vi "Standard Engine.vi"(8 "error in":errorcluster, 11 "Engine Process Init Data":T1) -> (0 "error out":errorcluster)   [LabVIEW 2013, in "Standard Engine Runtime.lvclass"]
doc: "This VI is a process that executes modules and has an API for transitioning through its state machine. Once it is initialized and running, it calls an array of module input methods, followed by an array of module process methods, followed by an array of module output methods, and then does any necessary error handling and bookkeeping."
uses:
  Standard Engine Runtime.lvclass
  Engine Process Init Data.ctl
  Commands.ctl
  Engine Config Data.ctl
  Configuration/Standard Engine Configuration.lvclass
  <vilib>/NI/Tag Bus Module Framework/runtime/TBM module execution interface.lvclass
  <vilib>/NI/Tag Bus Module Framework/module configuration/TBM module configuration.lvclass
  <vilib>/NI/Module Execution Interface/Engine Runtime/Execution States.ctl
  Engine Data.ctl
  Configuration/Loop Info.ctl
  <vilib>/NI/Tag Bus/table/data table.ctl
  Module Execution Info.ctl
  Data Table with Transfer Spec.ctl
  <vilib>/NI/Tag Bus/table/transfer specification.ctl
  <vilib>/NI/Tag Bus/tag/Data Type.ctl
  Configuration/Module Decimation.ctl
  Configuration/Module Error Configuration.ctl
  Configuration/Error Actions By Category.ctl
  <vilib>/NI/Tag Bus Module Framework/runtime/error classification.ctl
  Configuration/Error Actions.ctl
  <vilib>/NI/Module Timing Source/timing source/TBM timing source.lvclass
  Configuration/timing policy.ctl
  async execution info.ctl
  asynchronous process data.ctl
  async command notification.ctl
  <vilib>/NI/Tag Bus Module Framework/runtime/execution settings.ctl
  async error info.ctl
  status reporting data.ctl
  module status reporting.ctl
  <vilib>/Platform/TimedLoop/XDataNode/timing_clust.ctl
  <vilib>/Platform/TimedLoop/XDataNode/nitl_modes.ctl
  <vilib>/Platform/TimedLoop/XDataNode/wakeup.ctl
  <vilib>/NI/Tag Bus/table/transfer table data.vi
  Module Execution Decimation.vi
  Error Handler.vi
  <vilib>/NI/Tag Bus/table/write data element.vi
  <vilib>/NI/Tag Bus/table/data polymorphs/write one/write Boolean.vi
  <vilib>/NI/Tag Bus/table/data polymorphs/write one/write U32.vi
  <vilib>/NI/Tag Bus/table/data polymorphs/write one/write U64.vi
  <vilib>/NI/Tag Bus/table/data polymorphs/write one/write I32.vi
  Delete Module Index.vi
  <vilib>/platform/TimedLoop/XDataNode/XDataNode.xnode
  <vilib>/NI/Module Execution Interface/Engine Runtime/Engine Runtime Interface.lvclass
  <vilib>/NI/Tag Bus/table/data table.lvlib
  <vilib>/NI/Tag Bus/tag/tag descriptor.lvclass
  <vilib>/Platform/TimedLoop/XDataNode/XDNodeRunTimeDep.lvlib
panel:
  out "iterations":i32
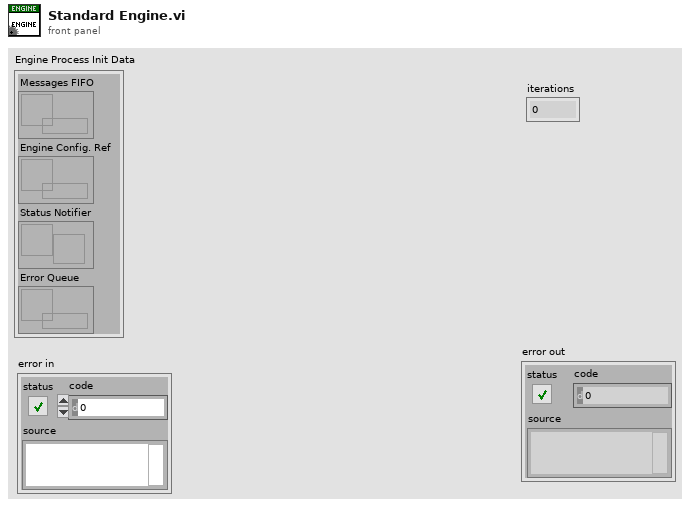
[diagram p1: front panel]
types:
  T1 = typedef "Standard Engine Runtime.lvclass/Engine Process Init Data.ctl" = cluster{"Messages FIFO":refnum<k33>, "Engine Config. Ref":refnum<data-value>, "Status Notifier":refnum<notifier>, "Error Queue":refnum<queue>}
  T2 = typedef "Standard Engine Runtime.lvclass/Engine Data.ctl" = cluster{"Loop Info":T3, "Main Tag Data":T4, "Module Info":T5, "engine timing source":refnum<class "TBM timing source.lvclass">, "timing policy":T14, "async execution info":T15, "status reporting":T18, "Timing Source dt":u32}
  T3 = typedef "Standard Engine Configuration.lvclass/Loop Info.ctl" = cluster{"Processor":i32, "Priority":i32}
  T4 = typedef "tag bus.lvlib/data table.lvlib/data table.ctl" = cluster{"Double":dbl[], "Single":sgl[], "I64":i64[], "I32":i32[], "I16":i16[], "I8":i8[], "U64":u64[], "U32":u32[], "U16":u16[], "U8":u8[], "Boolean":bool[], "String":string[], "Array of Double":cluster{"DBL Array":dbl[]}[], "Array of Single":cluster{"SGL Array":sgl[]}[], "Array of I64":cluster{"I64 Array":i64[]}[], "Array of I32":cluster{"I32 Array":i32[]}[], "Array of I16":cluster{"I16 Array":i16[]}[], "Array of I8":cluster{"I8 Array":i8[]}[], "Array of U64":cluster{"U64 Array":u64[]}[], "Array of U32":cluster{"U32 Array":u32[]}[], "Array of U16":cluster{"U16 Array":u16[]}[], "Array of U8":cluster{"U8 Array":u8[]}[], "Array of Boolean":cluster{"Boolean Array":bool[]}[], "Array of String":cluster{"String Array":string[]}[]}
  T5 = typedef "Standard Engine Runtime.lvclass/Module Execution Info.ctl" = cluster{"Tag Bus Modules":refnum<class "TBM module execution interface.lvclass">[], "Execute?":bool[], "Input Method Indices":i32[], "Process Method Indices":i32[], "Output Method Indices":i32[], "Input Transfer Specifications":T6[], "Parameter Transfer Specifications":T6[], "Result Transfer Specifications":T6[], "Output Transfer Specifications":T6[], "Module Errors":errorcluster[], "Module Decimation":T9[], "Module Decimation Indices":i32[], "Error Queue":refnum<queue>, "Module Error Configuration":T10[], "Module Errors (n-1)":errorcluster[]}
  T6 = typedef "Standard Engine Runtime.lvclass/Data Table with Transfer Spec.ctl" = cluster{"Data Table":T4, "Transfer Specification":T7[]}
  T7 = typedef "tag bus.lvlib/data table.lvlib/transfer specification.ctl" = cluster{"data type":T8, "sink indices":i32[], "source indices":i32[]}
  T8 = typedef "tag bus.lvlib/tag descriptor.lvclass/Data Type.ctl" = enum16{"Double", "Single", "I64", "I32", "I16", "I8", "U64", "U32", "U16", "U8", "Boolean", "String", "Array of Double", "Array of Single", "Array of I64", "Array of I32", "Array of I16", "Array of I8", "Array of U64", "Array of U32", "Array of U16", "Array of U8", "Array of Boolean", "Array of String"}
  T9 = typedef "Standard Engine Configuration.lvclass/Module Decimation.ctl" = cluster{"Decimation":u16, "Offset":u16}
  T10 = typedef "Standard Engine Configuration.lvclass/Module Error Configuration.ctl" = cluster{"Module Error Configuration":T11[]}
  T11 = typedef "Standard Engine Configuration.lvclass/Error Actions By Category.ctl" = cluster{"error classification":T12, "Error Actions":T13[]}
  T12 = typedef "TBM module execution interface.lvclass/error classification.ctl" = enum16{"unknown", "none", "trivial", "recoverable", "critical"}
  T13 = typedef "Standard Engine Configuration.lvclass/Error Actions.ctl" = enum16{"Clear", "Notify", "Stop Component", "Stop Engine", "Safe State", "Attempt Recovery"}
  T14 = typedef "Standard Engine Configuration.lvclass/timing policy.ctl" = enum16{"strict determinism", "nonblocking", "nondeterministic inline"}
  T15 = typedef "Standard Engine Runtime.lvclass/async execution info.ctl" = cluster{"Tag Bus Modules":T16[], "Execute?":bool[], "Input Method Indices":i32[], "Process Method Indices":i32[], "Output Method Indices":i32[], "Input Transfer Specifications":T6[], "Parameter Transfer Specifications":T6[], "Result Transfer Specifications":T6[], "Output Transfer Specifications":T6[], "Module Errors":errorcluster[], "Module Decimation":T9[], "Module Decimation Indices":i32[], "Error Queue":refnum<queue>, "Module Error Configuration":T10[], "comm errors":errorcluster[]}
  T16 = typedef "Standard Engine Runtime.lvclass/asynchronous process data.ctl" = cluster{"thread reference":refnum<vi>, "cmd notification":refnum<k33>, "execution period (ms)":i32, "input from component":refnum<queue>, "input to component":refnum<queue>, "output from component":refnum<queue>, "output to component":refnum<queue>, "process input from component":refnum<queue>, "process input to component":refnum<queue>, "process result from component":refnum<queue>, "process result to component":refnum<queue>, "execution settings":T17, "error fifo":refnum<k33>}
  T17 = typedef "TBM module execution interface.lvclass/execution settings.ctl" = cluster{"reads inputs":bool, "processes data":bool, "writes outputs":bool}
  T18 = typedef "Standard Engine Runtime.lvclass/status reporting data.ctl" = cluster{"late index (bool)":i32, "late count (U32)":i32, "current dt ns(U64)":i32, "synchronous modules":T19[], "asynchronous modules":T19[]}
  T19 = typedef "Standard Engine Runtime.lvclass/module status reporting.ctl" = cluster{"module index":i32, "error tag (I32)":i32}
  T20 = typedef "Engine Runtime Interface.lvclass/Execution States.ctl" = enum16{"Initializing", "Paused (Initialized)", "Running", "Set Safe Outputs", "Uninitializing", "Stopped (Uninitialized)", "Error (Uninitialized)", "Safe State (Uninitialized)", "Closed"}
  T21 = typedef "Standard Engine Runtime.lvclass/Commands.ctl" = enum16{"Initialize", "Start", "Pause", "Safe State", "Normal", "Stop", "Shutdown"}
  T22 = typedef "XDNodeRunTimeDep.lvlib/timing_clust.ctl" = cluster{"Expected End [f-1]":u64, "Actual End [f-1]":u64, "Finished Late? [f-1]":bool, "Expected End [i-1]":u64, "Actual End [i-1]":u64, "Finished Late? [i-1]":bool, "Expected Start [i]":u64, "Actual Start [i]":u64, "Expected Start [f]":u64, "Actual Start [f]":u64, "Source Name":string, "Structure Name":string, "Period":i64, "Deadline":i64, "Offset":i64, "Start":i64, "Priority":i32, "Timeout":i32, "Mode":T23, "Wakeup Reason":T24, "Error":errorcluster, "Source Type":string, "Secondary Source Type":string, "Global End Time":u64, "Global Start Time":u64, "Frame Duration":u64, "Iteration Duration":u64, "Assigned CPU":i32, "I/O Scan Engine Mode":u32}
  T23 = typedef "XDNodeRunTimeDep.lvlib/nitl_modes.ctl" = enum32{"No Change", "Process missed periods, maintain original phase", "Discard missed periods, maintain original phase", "Process missed periods, ignore original phase", "Discard missed periods, ignore original phase"}
  T24 = typedef "XDNodeRunTimeDep.lvlib/wakeup.ctl" = enum32{"Normal", "Aborted", "Asynchronous wakeup", "Timing source error", "Timed loop error", "Timeout"}
  T25 = typedef "Standard Engine Runtime.lvclass/Engine Config Data.ctl" = cluster{"Engine Configuration":refnum<class "Standard Engine Configuration.lvclass">, "Modules":refnum<class "TBM module execution interface.lvclass">[], "Module Configurations":refnum<class "TBM module configuration.lvclass">[]}
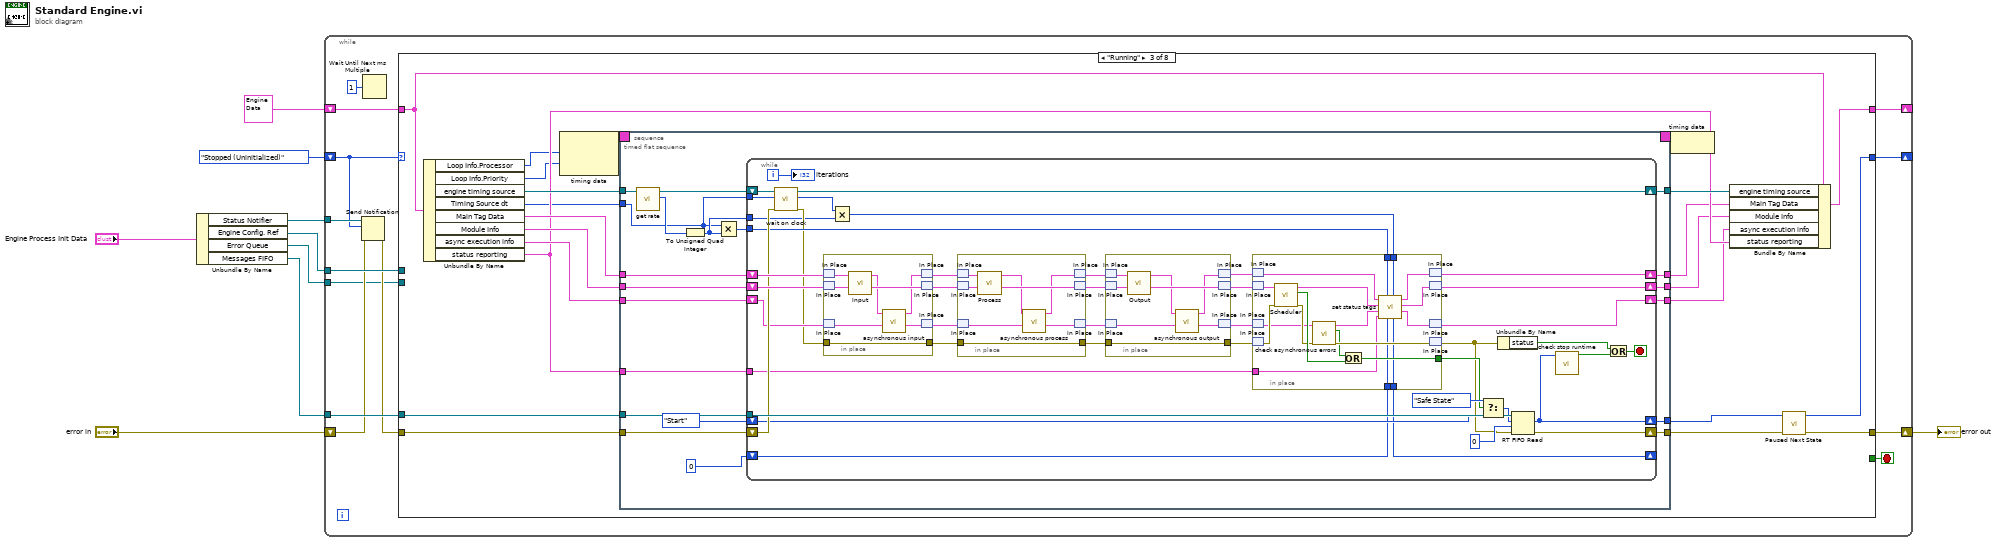
[diagram p0: block diagram]
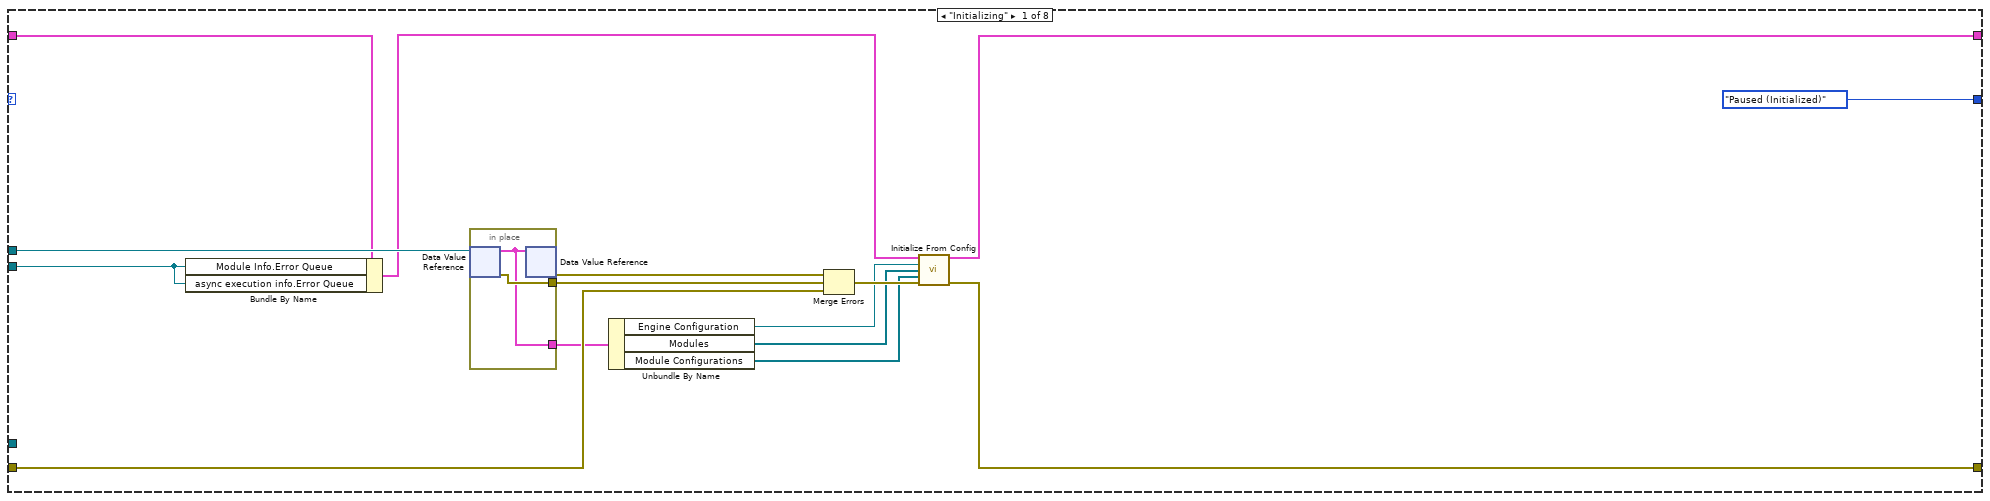
[diagram p2: hidden frame]
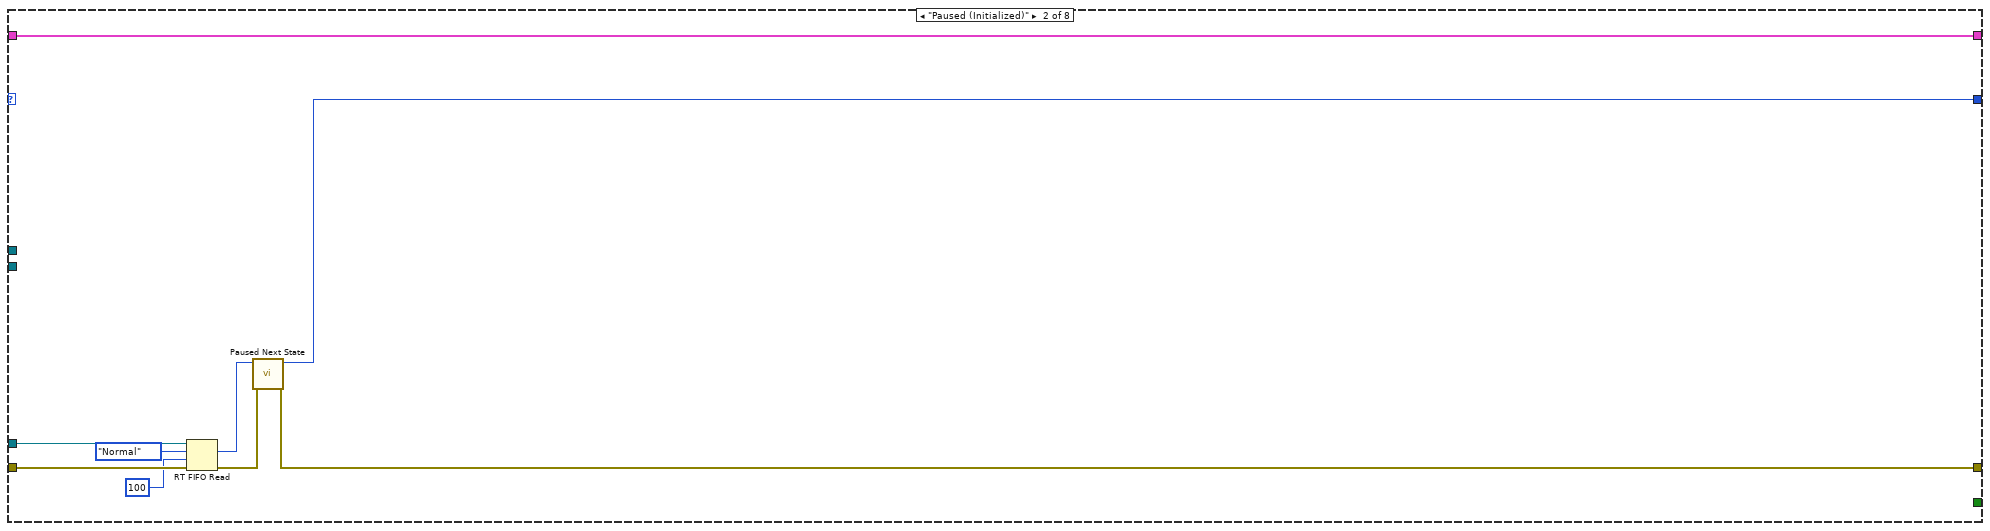
[diagram p3: hidden frame]
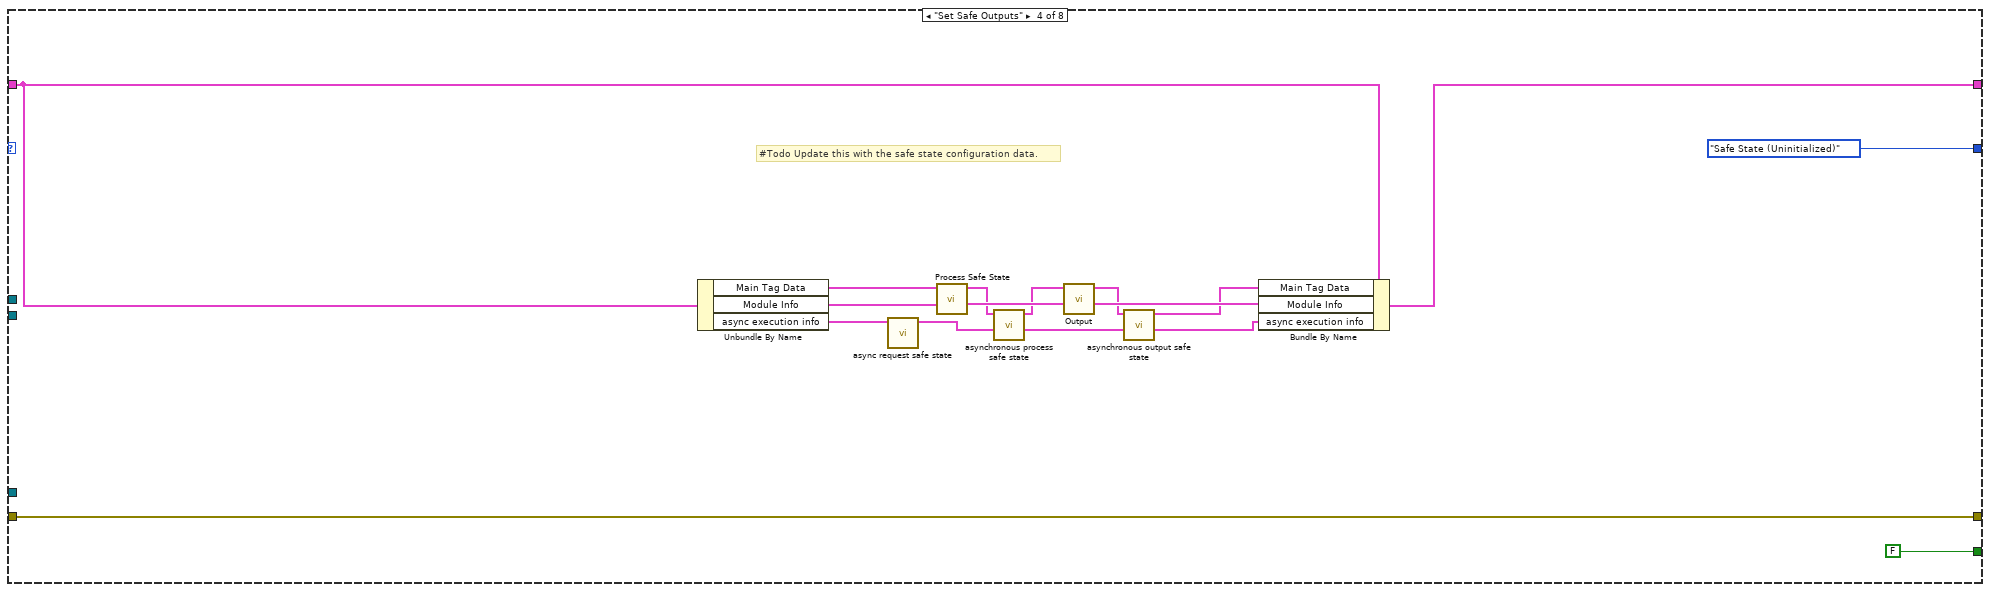
[diagram p4: hidden frame]
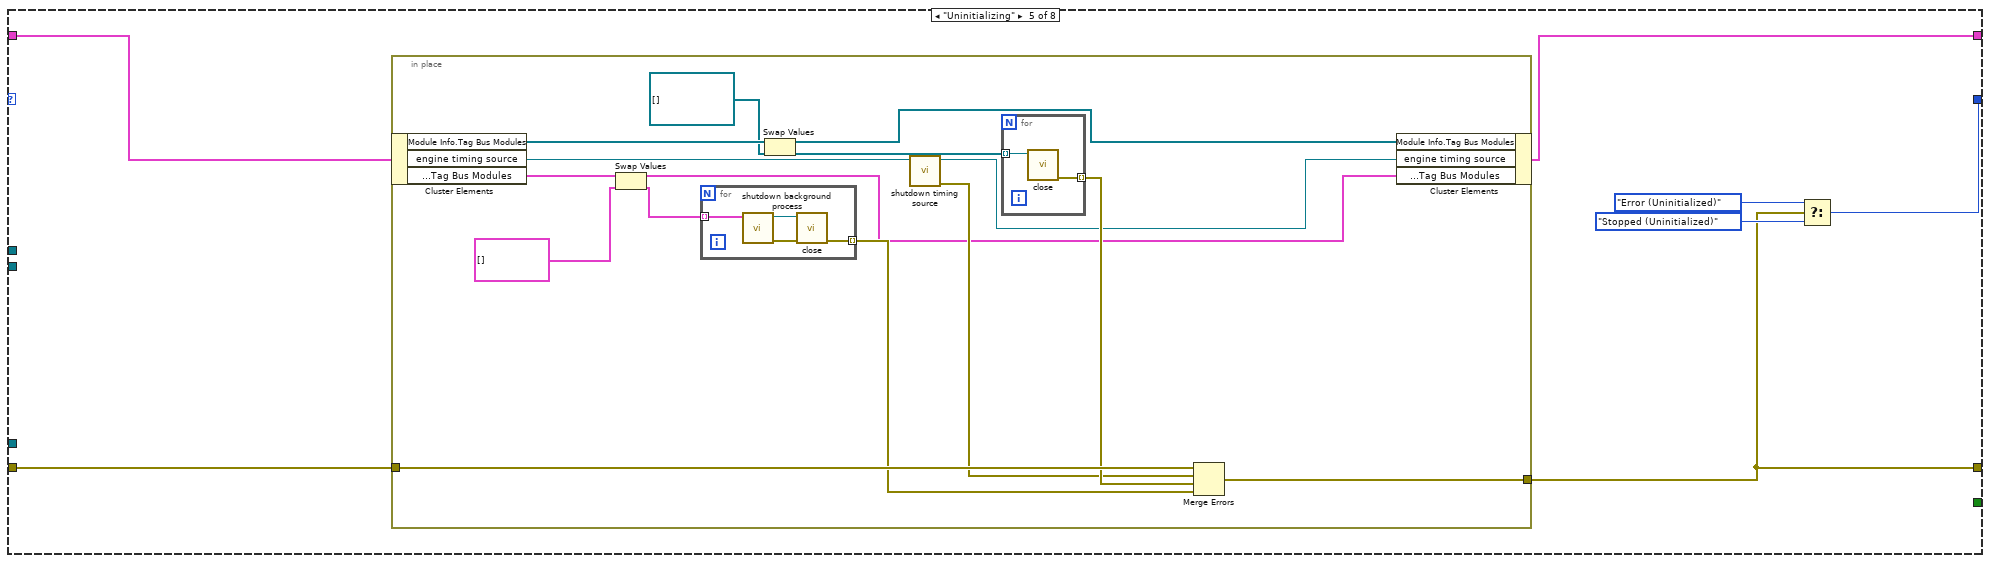
[diagram p5: hidden frame]
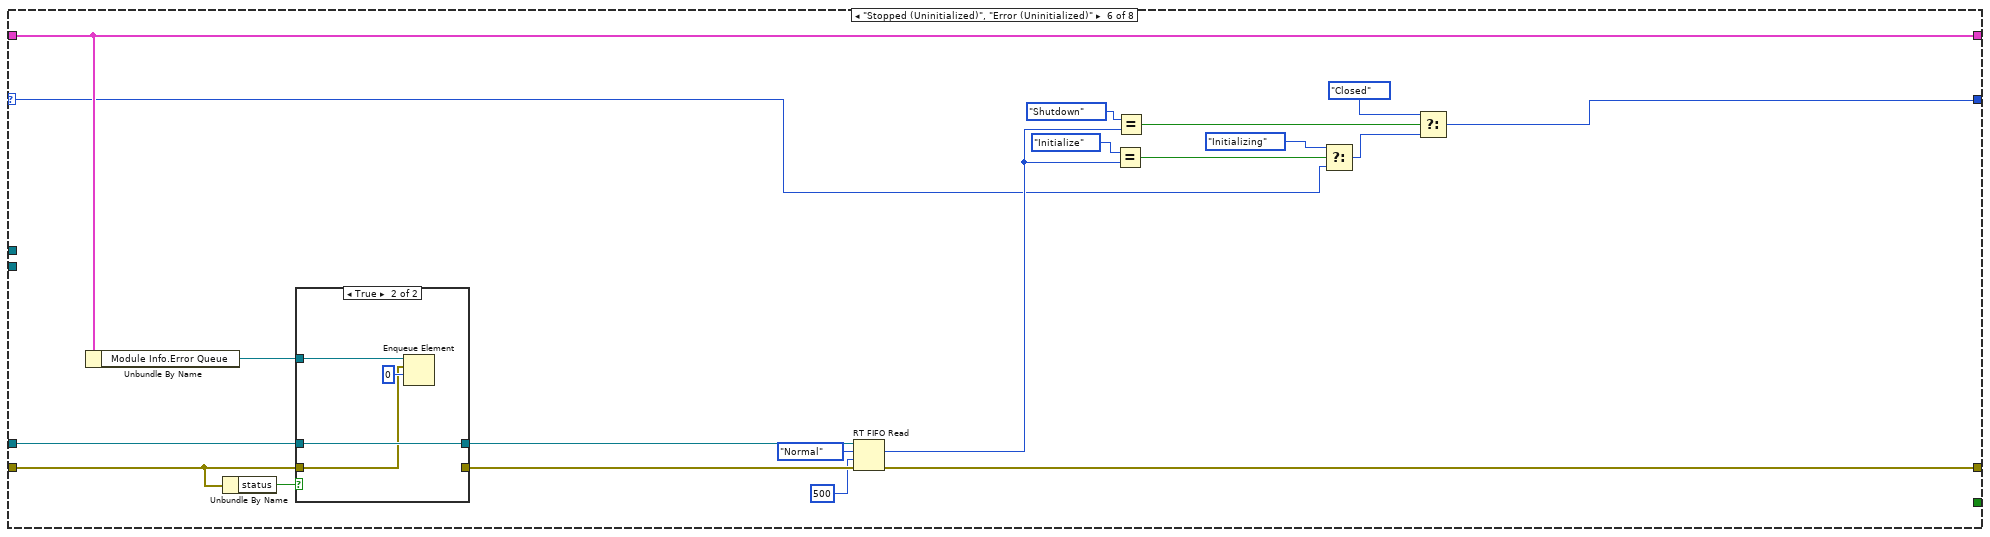
[diagram p6: hidden frame]
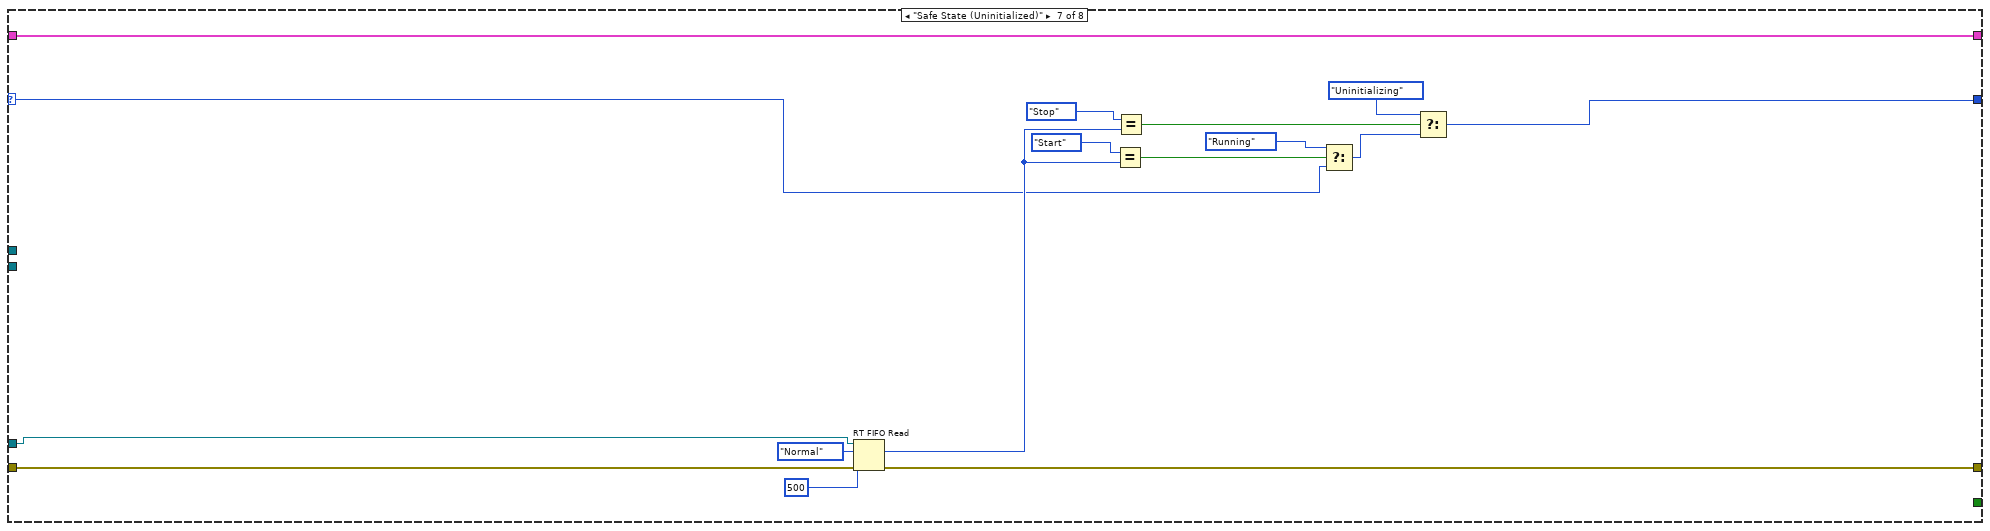
[diagram p8: hidden frame]
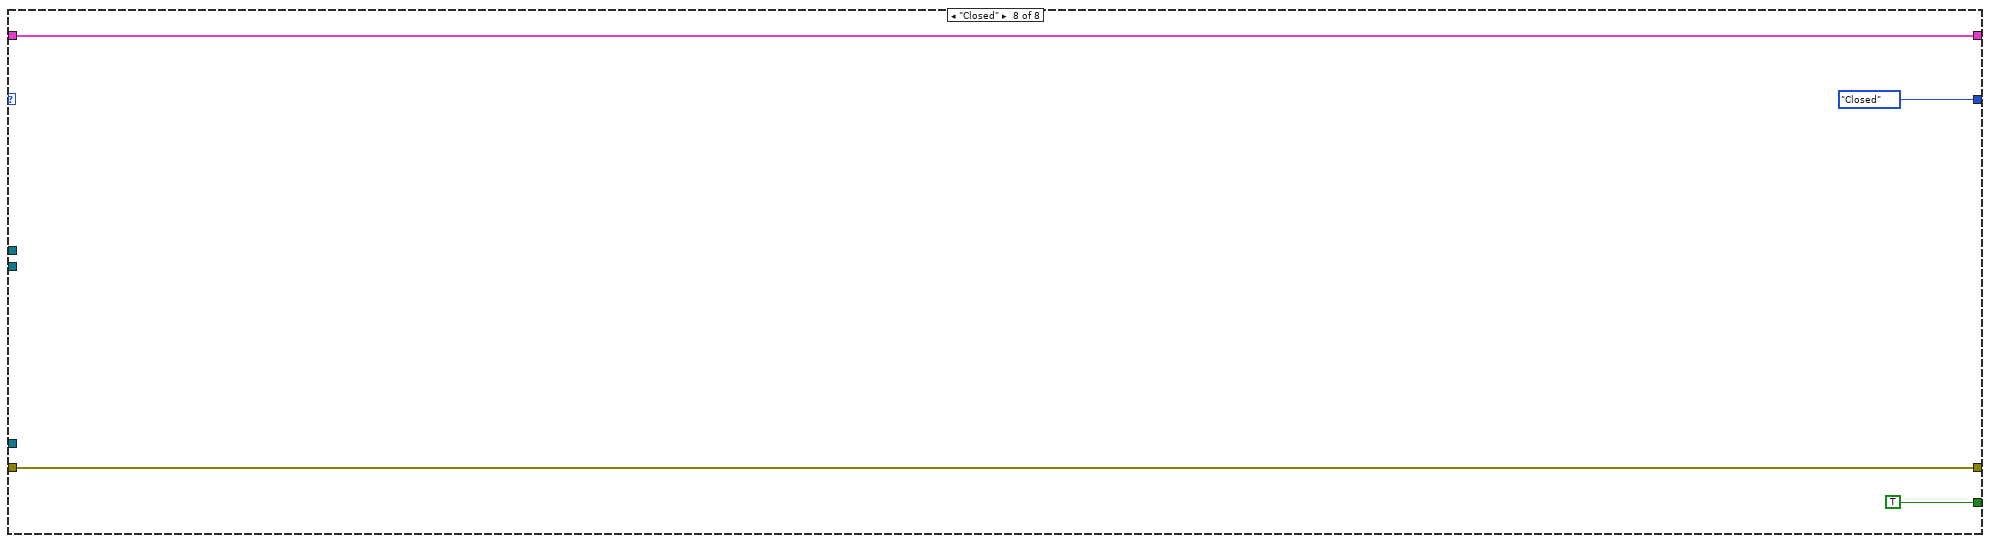
[diagram p9: hidden frame]
diagram:
  n1 = Unbundle By Name("Engine Process Init Data") -> ("Status Notifier"=w7:refnum<notifier>, "Engine Config. Ref"=w6:refnum<data-value>, "Error Queue"=w3:refnum<queue>, "Messages FIFO"=w5:refnum<k33>)
  n2 = while {
    shift-right: [w19] -> _
    shift-left: Execution_States."Stopped (Uninitialized)" ("States") -> [w14]
    shift-right: [w20] -> _
    shift-left: T2 {"Loop Info"={"Processor"=-2, "Priority"=0}, "Main Tag Data"={"Double"=[], "Single"=[], "I64"=[], "I32"=[], "I16"=[], "I8"=[], "U64"=[], "U32"=[], "U16"=[], "U8"=[], "Boolean"=[], "String"=[], "Array of Double"=[], "Array of Single"=[], "Array of I64"=[], "Array of I32"=[], "Array of I16"=[], "Array of I8"=[], "Array of U64"=[], "Array of U32"=[], "Array of U16"=[], "Array of U8"=[], "Array of Boolean"=[], "Array of String"=[]}, "Module Info"={"Tag Bus Modules"=[], "Execute?"=[], "Input Method Indices"=[], "Process Method Indices"=[], "Output Method Indices"=[], "Input Transfer Specifications"=[], "Parameter Transfer Specifications"=[], "Result Transfer Specifications"=[], "Output Transfer Specifications"=[], "Module Errors"=[], "Module Decimation"=[], "Module Decimation Indices"=[], "Error Queue"=refnum, "Module Error Configuration"=[], "Module Errors (n-1)"=[]}, "engine timing source"=refnum, "timing policy"=enum."nonblocking", "async execution info"={"Tag Bus Modules"=[], "Execute?"=[], "Input Method Indices"=[], "Process Method Indices"=[], "Output Method Indices"=[], "Input Transfer Specifications"=[], "Parameter Transfer Specifications"=[], "Result Transfer Specifications"=[], "Output Transfer Specifications"=[], "Module Errors"=[], "Module Decimation"=[], "Module Decimation Indices"=[], "Error Queue"=refnum, "Module Error Configuration"=[], "comm errors"=[]}, "status reporting"={"late index (bool)"=0, "late count (U32)"=0, "current dt ns(U64)"=0, "synchronous modules"=[], "asynchronous modules"=[]}, "Timing Source dt"=0} ("Engine Data Out") -> [w22]
    shift-right: [w21] -> w8
    shift-left: "error in" -> [w13]
    tunnel: w5 -> [w18]
    tunnel: w6 -> [w16]
    tunnel: w7 -> [w15]
    tunnel: w3 -> [w11]
    stop <- w17 stop-if-true
    n3 = Send Notification(notification=w14, notifier=w15, error in (no error)=w13) -> (error out=w12:errorcluster)  [unwired: 1 out]
    n4 = Wait Until Next ms Multiple(millisecond multiple=u32 1) -> ()  [unwired: 1 out]
    n5 = case shown="\"Running\"" w14 {
      selector: w14 -> [_ _ _ _ _ w247 w271 _]
      tunnel: w22 -> [w26 w48 w68 w210 w216 w249 w272 w286]
      tunnel: w12 -> [w34 w47 w54 w214 w218 w243 w274 w288]
      tunnel: [w24 w42 w66 w214 w217 w258 w281 w288] -> w21
      tunnel: [w32 w48 w67 w211 w215 w249 w272 w286] -> w20
      tunnel: [Execution_States."Paused (Initialized)" ("States") w46 w69 Execution_States."Safe State (Uninitialized)" ("States") w219 w259 w282 Execution_States."Closed" ("States")] -> w19
      tunnel: w18 -> [_ w41 w70 _ _ w251 w273 _]
      tunnel: [_ _ _ FALSE _ _ _ TRUE] -> w17
      tunnel: w16 -> [w29 _ _ _ _ _ _ _]
      tunnel: w11 -> [w23 _ _ _ _ _ _ _]
      frame "Initializing" {
        n6 = Bundle By Name(cluster=w26, "Module Info.Error Queue"=w23, "async execution info.Error Queue"=w23) -> (w25:T2)
        n7 = in-place {
          in-place-border: [w39] -> w35
          in-place-border: [w38] -> w33
          n8 = in-place-dvr #1(w29) -> (w38:T25, w39:errorcluster)
          n9 = in-place-dvr #1(w38) -> (w36:errorcluster)  [unwired: 1 out]
        }
        n10 = Unbundle By Name(w33) -> ("Engine Configuration"=w30:refnum<class "Standard Engine Configuration.lvclass">, "Modules"=w28:refnum<class "TBM module execution interface.lvclass">[], "Module Configurations"=w27:refnum<class "TBM module configuration.lvclass">[])
        n11 = Merge Errors(w36, w35, w34) -> (w31:errorcluster)
        n12 = call "Initialize From Config.vi"("Engine Data"=w25, "Engine Configuration"=w30, "Modules"=w28, "Module Configurations"=w27, "error in"=w31) -> ("Engine Data Out"=w32:T2, "error out"=w24:errorcluster)  [unwired: 9 in]
      }
      frame "Paused (Initialized)" {
        n13 = RT FIFO Read(0:w41, 1:Commands."Normal" ("Commands"), 2:100 ("timeout in ms (0)"), 3:w47) -> (9:w45:T21, 11:w44:errorcluster)  [unwired: 3 out]
        n14 = call "Paused Next State.vi"("error in"=w44, "Command"=w45) -> ("error out"=w42:errorcluster, "State"=w46:T20)  [unwired: 8 in]
      }
      frame "Running" {
        n15 = Unbundle By Name(w68) -> ("Loop Info.Processor"=w51:i32, "Loop Info.Priority"=w50:i32, "engine timing source"=w63:refnum<class "TBM timing source.lvclass">, "Timing Source dt"=w49:u32, "Main Tag Data"=w62:T4, "Module Info"=w61:T5, "async execution info"=w60:T15, "status reporting"=w58:T18)
        n16 = node-c288(w51, w50) -> (w53:T22)
        n17 = timed-sequence {
          timing: w53 -> [_]
          timing-out: [_] -> w52
          tunnel: w70 -> [w84]
          tunnel: [w83] -> w65
          tunnel: [w82] -> w64
          tunnel: w63 -> [w72]
          tunnel: w62 -> [w81]
          tunnel: w61 -> [w80]
          tunnel: w60 -> [w79]
          tunnel: [w78] -> w59
          tunnel: w58 -> [w77]
          tunnel: [w76] -> w57
          tunnel: [w75] -> w56
          tunnel: [w74] -> w55
          tunnel: w54 -> [w73]
          tunnel: w49 -> [w71]
          n18 = timed-flat-sequence {
            tunnel: w84 -> [w104]
            tunnel: [w103] -> w83
            tunnel: [w102] -> w82
            tunnel: w81 -> [w101]
            tunnel: w80 -> [w100]
            tunnel: w79 -> [w99]
            tunnel: [w98] -> w78
            tunnel: w77 -> [w97]
            tunnel: [w96] -> w76
            tunnel: [w95] -> w75
            tunnel: [w94] -> w74
            tunnel: w73 -> [w90]
            tunnel: w72 -> [w89]
            tunnel: w71 -> [w85]
            n19 = call-dynamic "get rate.vi"("timing source in"=w89) -> ("period (ns)"=w87:i64, "timing source out"=w92:refnum<class "TBM timing source.lvclass">)  [unwired: 8 in, 1 out]
            n20 = To Unsigned Quad Integer(1:w87) -> (0:w86:u64)
            n21 = Multiply(x=w85, y=w86) -> (x*y=w88:u64)
            n22 = while {
              tunnel: w104 -> [w137]
              shift-right: [w139] -> w103
              shift-left: Commands."Start" ("Commands") -> [w125]
              shift-right: [w119] -> w96
              shift-left: w101 -> [w146]
              shift-right: [w140] -> w95
              shift-left: w100 -> [w145]
              shift-right: [w136] -> w102
              shift-left: w90 -> [w132]
              shift-right: [w131] -> w98
              shift-left: w92 -> [w133]
              tunnel: w88 -> [w118]
              shift-right: [w126] -> w94
              shift-left: w99 -> [w130]
              tunnel: w97 -> [w117]
              shift-right: [w116] -> _
              shift-left: u32 0 ("late count out") -> [w115]
              tunnel: w86 -> [w110]
              tunnel: w85 -> [w105]
              i -> [w135]
              stop <- w107 stop-if-true
              n23 = call-dynamic "wait on clock.vi"("error in"=w132, "dt"=w105, "timing source in"=w133) -> ("error out"=w114:errorcluster, "ticks since last call"=w109:u32, "timing source out"=w131:refnum<class "TBM timing source.lvclass">)  [unwired: 6 in]
              n24 = in-place {
                in-place-border: w114 -> [w186]
                in-place-border: [w186] -> w111
                n25 = in-place-match #2(w146) -> (w185:T4)
                n26 = in-place-match #3(w145) -> (w190:T5)
                n27 = in-place-match #4(w130) -> (w188:T15)
                n28 = call "Input.vi"("Module Info In"=w190, "Engine Tags In"=w185) -> ("Module Info Out"=w189:T5, "Engine Tags Out"=w184:T4)  [unwired: 8 in]
                n29 = call "asynchronous input.vi"("Module Info In"=w188, "Engine Tags In"=w184) -> ("Module Info Out"=w187:T15, "Engine Tags Out"=w183:T4)  [unwired: 8 in]
                n30 = in-place-match #2(w183) -> (w144:T4)
                n31 = in-place-match #3(w189) -> (w143:T5)
                n32 = in-place-match #4(w187) -> (w129:T15)
              }
              n33 = Multiply(x=w109, y=w110) -> (x*y=w108:u64)
              n34 = in-place {
                in-place-border: [w175] -> w112
                in-place-border: w111 -> [w175]
                n35 = in-place-match #5(w144) -> (w181:T4)
                n36 = in-place-match #6(w143) -> (w182:T5)
                n37 = in-place-match #7(w129) -> (w179:T15)
                n38 = call "Process.vi"("Module Info In"=w182, "Engine Tags In"=w181) -> ("Module Info Out"=w180:T5, "Engine Tags Out"=w178:T4)  [unwired: 8 in]
                n39 = call "asynchronous process.vi"("Module Info In"=w179, "Engine Tags In"=w178) -> ("Module Info Out"=w177:T15, "Engine Tags Out"=w176:T4)  [unwired: 8 in]
                n40 = in-place-match #5(w176) -> (w134:T4)
                n41 = in-place-match #6(w180) -> (w142:T5)
                n42 = in-place-match #7(w177) -> (w128:T15)
              }
              n43 = in-place {
                in-place-border: [w167] -> w113
                in-place-border: w112 -> [w167]
                n44 = in-place-match #8(w134) -> (w174:T4)
                n45 = in-place-match #9(w142) -> (w173:T5)
                n46 = in-place-match #10(w128) -> (w171:T15)
                n47 = call "Output.vi"("Module Info In"=w173, "Engine Tags In"=w174) -> ("Module Info Out"=w172:T5, "Engine Tags Out"=w169:T4)  [unwired: 8 in]
                n48 = call "asynchronous output.vi"("Module Info In"=w171, "Engine Tags In"=w169) -> ("Module Info Out"=w170:T15, "Engine Tags Out"=w168:T4)  [unwired: 8 in]
                n49 = in-place-match #8(w168) -> (w120:T4)
                n50 = in-place-match #9(w172) -> (w141:T5)
                n51 = in-place-match #10(w170) -> (w127:T15)
              }
              n52 = in-place {
                in-place-border: [w162] -> w122
                in-place-border: w118 -> [w149]
                in-place-border: w108 -> [w148]
                in-place-border: w117 -> [w150]
                in-place-border: [w152] -> w116
                in-place-border: w115 -> [w151]
                n53 = in-place-match #11(w120) -> (w158:T4)
                n54 = in-place-match #12(w141) -> (w159:T5)
                n55 = in-place-match #13(w127) -> (w160:T15)
                n56 = in-place-match #14(w113) -> (w166:errorcluster)
                n57 = call "Scheduler.vi"("error in"=w166, "Module Info In"=w159) -> ("error out"=w164:errorcluster, "Safe State?"=w165:bool, "Module Info Out"=w157:T5)  [unwired: 7 in]
                n58 = call "check asynchronous errors.vi"("error in"=w164, "Module Info In"=w160) -> ("error out"=w163:errorcluster, "safe state?"=w161:bool, "Module Info Out"=w154:T15)  [unwired: 7 in]
                n59 = Or(x=w161, y=w165) -> (x .or. y?=w162:bool)
                n60 = call "set status tags.vi"("ns since last call"=w148, "late count in"=w151, "desired dt ns"=w149, "status reporting"=w150, "async module info in"=w154, "Module Info In"=w157, "Engine Tags In"=w158) -> ("async module info out"=w153:T15, "Module Info Out"=w155:T5, "Engine Tags Out"=w156:T4, "late count out"=w152:u32)  [unwired: 1 in]
                n61 = in-place-match #11(w156) -> (w119:T4)
                n62 = in-place-match #12(w155) -> (w140:T5)
                n63 = in-place-match #13(w153) -> (w126:T15)
                n64 = in-place-match #14(w163) -> (w121:errorcluster)
              }
              n65 = Select(t=Commands."Safe State" ("y"), s=w122, f=w125) -> (s? t:f=w124:T21)
              n66 = Unbundle By Name(w121) -> ("status"=w106:bool)
              n67 = RT FIFO Read(0:w137, 1:w124, 2:0 ("timeout in ms (0)"), 3:w121) -> (9:w139:T21, 11:w136:errorcluster)  [unwired: 3 out]
              n68 = call "check stop runtime.vi"("Commands"=w139) -> ("stop?"=w138:bool)  [unwired: 10 in]
              n69 = Or(x=w106, y=w138) -> (x .or. y?=w107:bool)
              "iterations" <- w135
            }
          }
        }
        n70 = node-c288(w52) -> ()
        n71 = Bundle By Name(cluster=w68, "engine timing source"=w59, "Main Tag Data"=w57, "Module Info"=w56, "async execution info"=w55, "status reporting"=w58) -> (w67:T2)
        n72 = call "Paused Next State.vi"("error in"=w64, "Command"=w65) -> ("error out"=w66:errorcluster, "State"=w69:T20)  [unwired: 8 in]
      }
      frame "Set Safe Outputs" {
        # "#Todo Update this with the safe state configuration data."
        n73 = Unbundle By Name(w210) -> ("Main Tag Data"=w209:T4, "Module Info"=w208:T5, "async execution info"=w202:T15)
        n74 = call "async request safe state.vi"("async execution info in"=w202) -> ("async execution info out"=w203:T15)  [unwired: 10 in]
        n75 = call "Process Safe State.vi"("Module Info In"=w208, "Engine Tags In"=w209) -> ("Module Info Out"=w207:T5, "Engine Tags Out"=w205:T4)  [unwired: 8 in]
        n76 = call "asynchronous process safe state.vi"("Module Info In"=w203, "Engine Tags In"=w205) -> ("Module Info Out"=w198:T15, "Engine Tags Out"=w204:T4)  [unwired: 8 in]
        n77 = call "Output.vi"("Module Info In"=w207, "Engine Tags In"=w204) -> ("Module Info Out"=w206:T5, "Engine Tags Out"=w201:T4)  [unwired: 8 in]
        n78 = call "asynchronous output safe state.vi"("Module Info In"=w198, "Engine Tags In"=w201) -> ("Module Info Out"=w199:T15, "Engine Tags Out"=w200:T4)  [unwired: 8 in]
        n79 = Bundle By Name(cluster=w210, "Main Tag Data"=w200, "Module Info"=w206, "async execution info"=w199) -> (w211:T2)
      }
      frame "Uninitializing" {
        n80 = in-place {
          in-place-border: w218 -> [w236]
          in-place-border: [w235] -> w217
          n81 = in-place-cluster #15(w216) -> ("Module Info.Tag Bus Modules"=w225:refnum<class "TBM module execution interface.lvclass">[], "engine timing source"=w231:refnum<class "TBM timing source.lvclass">, "async execution info.Tag Bus Modules"=w230:T16[])
          n82 = Swap Values(12:w230, 14:T16[] []) -> (1:w227:T16[], 3:w229:T16[])  [unwired: 1 in]
          n83 = for {
            tunnel: [w238] -> w232 mode=indexing
            tunnel: w229 -> [w237] mode=indexing
            n84 = call "shutdown background process.vi"("async data"=w237) -> ("error out"=w240:errorcluster, "module out"=w239:refnum<class "TBM module execution interface.lvclass">)  [unwired: 8 in, 1 out]
            n85 = call-dynamic "close.vi"("error in"=w240, "module in"=w239) -> ("error out"=w238:errorcluster)  [unwired: 9 in]
          }
          n86 = Swap Values(12:w225, 14:refnum<class "TBM module execution interface.lvclass">[] [] ("y'")) -> (1:w223:refnum<class "TBM module execution interface.lvclass">[], 3:w224:refnum<class "TBM module execution interface.lvclass">[])  [unwired: 1 in]
          n87 = call-dynamic "shutdown timing source.vi"("timing source in"=w231) -> ("error out"=w233:errorcluster, "timing source out"=w226:refnum<class "TBM timing source.lvclass">)  [unwired: 9 in]
          n88 = for {
            tunnel: w224 -> [w242] mode=indexing
            tunnel: [w241] -> w234 mode=indexing
            n89 = call-dynamic "close.vi"("module in"=w242) -> ("error out"=w241:errorcluster)  [unwired: 10 in]
          }
          n90 = Merge Errors(w236, w233, w234, w232) -> (w235:errorcluster)
          n91 = in-place-cluster #15("Module Info.Tag Bus Modules"=w223, "engine timing source"=w226, "async execution info.Tag Bus Modules"=w227) -> (w215:T2)
        }
        n92 = Select(t=Execution_States."Error (Uninitialized)" ("States"), s=w217, f=Execution_States."Stopped (Uninitialized)" ("States")) -> (s? t:f=w219:T20)
      }
      frame "Stopped (Uninitialized)", "Error (Uninitialized)" {
        n93 = Unbundle By Name(w249) -> ("Module Info.Error Queue"=w248:refnum<queue>)
        n94 = Unbundle By Name(w243) -> ("status"=w244:bool)
        n95 = case shown="True" w244 {
          tunnel: w251 -> [w264 w268]
          tunnel: [w264 w268] -> w250
          tunnel: [w263 _] -> w246
          tunnel: w248 -> [_ w267]
          tunnel: w243 -> [w263 w265]
          frame False {
          }
          frame True {
            n96 = Enqueue Element(queue=w267, element=w265, timeout in ms (-1)=0) -> ()  [unwired: 1 in, 3 out]
          }
        }
        n97 = RT FIFO Read(0:w250, 1:Commands."Normal" ("Commands"), 2:500 ("milliseconds to wait"), 3:w246) -> (9:w262:T21, 11:w258:errorcluster)  [unwired: 3 out]
        n98 = Equal?(x=Commands."Initialize" ("Commands"), y=w262) -> (x = y?=w261:bool)
        n99 = Equal?(x=Commands."Shutdown" ("Commands"), y=w262) -> (x = y?=w257:bool)
        n100 = Select(t=Execution_States."Initializing" ("States"), s=w261, f=w247) -> (s? t:f=w260:T20)
        n101 = Select(t=Execution_States."Closed" ("States"), s=w257, f=w260) -> (s? t:f=w259:T20)
      }
      frame "Safe State (Uninitialized)" {
        n102 = RT FIFO Read(0:w273, 1:Commands."Normal" ("Commands"), 2:500 ("timeout in ms (0)"), 3:w274) -> (9:w284:T21, 11:w281:errorcluster)  [unwired: 3 out]
        n103 = Equal?(x=Commands."Start" ("Commands"), y=w284) -> (x = y?=w269:bool)
        n104 = Equal?(x=Commands."Stop" ("Commands"), y=w284) -> (x = y?=w280:bool)
        n105 = Select(t=Execution_States."Running" ("States"), s=w269, f=w271) -> (s? t:f=w283:T20)
        n106 = Select(t=Execution_States."Uninitializing" ("States"), s=w280, f=w283) -> (s? t:f=w282:T20)
      }
      frame "Closed" {
      }
    }
  }
  "error out" <- w8
